vi "Run.vi"(8 "error in (no error)":errorcluster, 11 "DaqMx_Single in":refnum<class "DaqMx_Single.lvclass">) -> (0 "error out":errorcluster, 3 "DaqMx_Single out":refnum<class "DaqMx_Single.lvclass">)   [LabVIEW 2014, in "FgenPlugins.lvlib" / "DaqMx_Single.lvclass"]
uses:
  DaqMx_Single.lvclass
  FgenPluginBaseClass/FgenPluginsBase.lvclass/FgenPluginsBase.ctl
  FgenPluginBaseClass/Accessors/Read FunctionClass.vi
  FgenPluginBaseClass/Accessors/Write FunctionClass.vi
  FgenPluginBaseClass/Accessors/Read Channels.vi
  MemberClasses/FunctionBaseClass/FunctionBase.lvclass
  FgenPluginBaseClass/FgenPluginsBase.lvclass
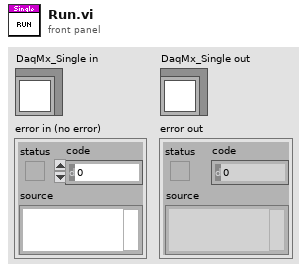
[diagram p1: front panel]
types:
  T1 = typedef "FgenPlugins.lvlib/DaqMx_Single.lvclass/clEvents.ctl" = cluster{"Stop":refnum<user-event>, "Params":refnum<user-event>}
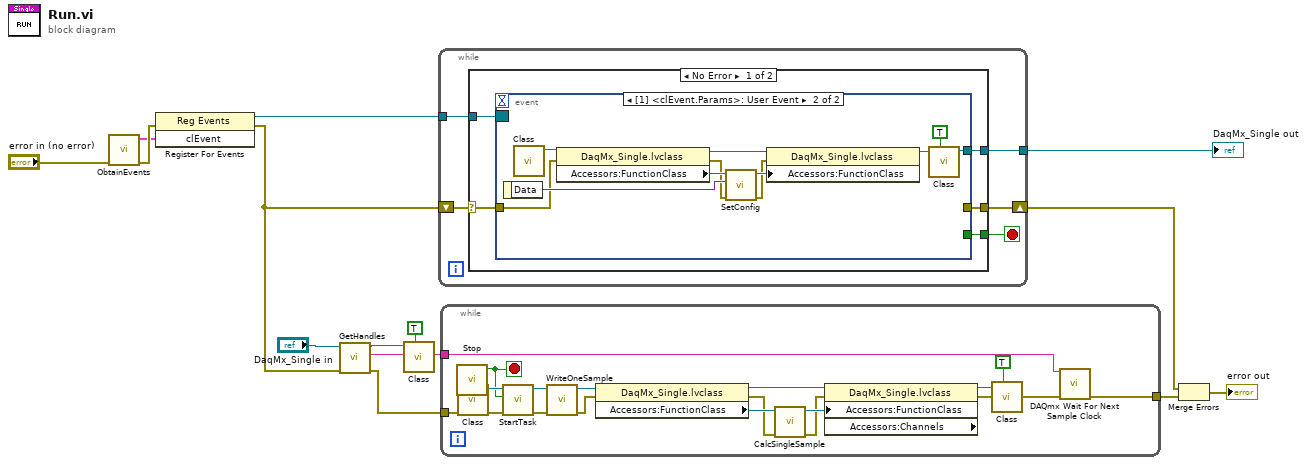
[diagram p0: block diagram]
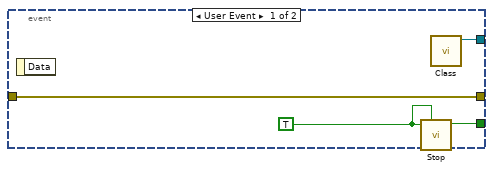
[diagram p2: hidden frame]
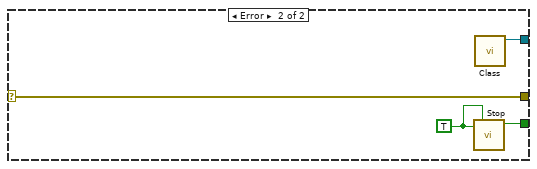
[diagram p3: hidden frame]
diagram:
  n1 = call "ObtainEvents.vi"("error in (no error)"="error in (no error)") -> ("error out"=w13:errorcluster, "clEvent"=w11:T1)  [unwired: 9 in]
  n2 = register-events(error in=w13, w11) -> (reference out=w14:refnum<event-registration>, error out=w2:errorcluster)  [unwired: 1 in]
  n3 = call "GetHandles.vi"("error in (no error)"=w2, "FgenPluginsBase in"="DaqMx_Single in") -> ("error out"=w1:errorcluster, "FirstHandle"=w3:string, "FgenPluginsBase out"=w4:refnum<class "DaqMx_Single.lvclass">)  [unwired: 6 in, 1 out]
  n4 = call "Class.vi"("Set? (f)"=TRUE, "DaqMx_Single in"=w4) -> ()  [unwired: 9 in, 1 out]
  n5 = while {
    tunnel: w14 -> [w19]
    tunnel: [w15] -> w10
    shift-right: [w16] -> w8
    shift-left: w2 -> [w17]
    stop <- w18 stop-if-true
    n6 = case shown="No Error" w17 {
      selector: w17 -> [w22 w41]
      tunnel: w19 -> [w24 _]
      tunnel: [w23 w42] -> w18
      tunnel: [w21 w41] -> w16
      tunnel: [w20 w40] -> w15
      frame No Error {
        n7 = event shown="[1] <clEvent.Params>: User Event" {
          selector: w24 -> [_ _]
          dyn-events: _ -> [_ _]
          timeout: _ -> [_ _]
          tunnel: [w27 _] -> w23
          tunnel: w22 -> [w26 w33]
          tunnel: [w26 _] -> w21
          tunnel: [w25 w29] -> w20
          event User Event {
            w28 = TRUE
            n8 = event-data() -> ()  [unwired: 1 in, 1 out]
            n9 = call "Stop.vi"("Set? (f)"=w28, "In"=w28) -> ("Out"=w27:bool)  [unwired: 9 in]
            n10 = call "Class.vi"() -> ("DaqMx_Single out"=w25:refnum<class "DaqMx_Single.lvclass">)  [unwired: 11 in]
          }
          event User Event {
            n11 = event-data() -> ("Data"=w37:variant)  [unwired: 1 in]
            n12 = call "Class.vi"() -> ("DaqMx_Single out"=w39:refnum<class "DaqMx_Single.lvclass">)  [unwired: 11 in]
            n13 = property class="DaqMx_Single.lvclass"(reference=w39, error in=w33) -> (reference out=w35:refnum<class "DaqMx_Single.lvclass">, error out=w32:errorcluster, "Accessors:FunctionClass"=w38:refnum<class "FunctionBase.lvclass">)
            n14 = call-dynamic "SetConfig.vi"("error in (no error)"=w32, "Variant"=w37, "FunctionBase in"=w38) -> ("error out"=w34:errorcluster, "FunctionBase out"=w36:refnum<class "FunctionBase.lvclass">)  [unwired: 7 in]
            n15 = property class="DaqMx_Single.lvclass"(reference=w35, error in=w34, "Accessors:FunctionClass"=w36) -> (reference out=w31:refnum<class "DaqMx_Single.lvclass">)  [unwired: 1 out]
            n16 = call "Class.vi"("Set? (f)"=TRUE, "DaqMx_Single in"=w31) -> ("DaqMx_Single out"=w29:refnum<class "DaqMx_Single.lvclass">)  [unwired: 9 in]
          }
        }
      }
      frame Error {
        w43 = TRUE
        n17 = call "Stop.vi"("Set? (f)"=w43, "In"=w43) -> ("Out"=w42:bool)  [unwired: 9 in]
        n18 = call "Class.vi"() -> ("DaqMx_Single out"=w40:refnum<class "DaqMx_Single.lvclass">)  [unwired: 11 in]
      }
    }
  }
  "DaqMx_Single out" <- w10
  n19 = while {
    tunnel: [w45] -> w7
    tunnel: w3 -> [w46]
    tunnel: w1 -> [w44]
    stop <- w48 stop-if-true
    n20 = call "Stop.vi"() -> ("Out"=w48:bool)  [unwired: 11 in]
    n21 = call "Class.vi"() -> ("DaqMx_Single out"=w49:refnum<class "DaqMx_Single.lvclass">)  [unwired: 11 in]
    n22 = call-dynamic "StartTask.vi"("error in (no error)"=w44, "Stop?"=w48, "DaqMx_Single in"=w49) -> ("error out"=w53:errorcluster, "DaqMx_Single out"=w52:refnum<class "DaqMx_Single.lvclass">)  [unwired: 7 in]
    n23 = call "WriteOneSample.vi"("error in (no error)"=w53, "DaqMx_Single in"=w52) -> ("error out"=w50:errorcluster, "DaqMx_Single out"=w51:refnum<class "DaqMx_Single.lvclass">)  [unwired: 8 in]
    n24 = property class="DaqMx_Single.lvclass"(reference=w51, error in=w50) -> (reference out=w58:refnum<class "DaqMx_Single.lvclass">, error out=w59:errorcluster, "Accessors:FunctionClass"=w60:refnum<class "FunctionBase.lvclass">)
    n25 = call-dynamic "CalcSingleSample.vi"("error in (no error)"=w59, "FunctionBase in"=w60) -> ("error out"=w56:errorcluster, "FunctionBase out"=w57:refnum<class "FunctionBase.lvclass">)  [unwired: 8 in]
    n26 = property class="DaqMx_Single.lvclass" props=["Accessors:FunctionClass", "Accessors:Channels"](reference=w58, error in=w56, "Accessors:FunctionClass"=w57) -> (reference out=w55:refnum<class "DaqMx_Single.lvclass">, error out=w47:errorcluster)  [unwired: 1 out]
    n27 = call "Class.vi"("Set? (f)"=TRUE, "DaqMx_Single in"=w55) -> ()  [unwired: 9 in, 1 out]
    n28 = call <vilib>:"DAQmx Wait For Next Sample Clock.vi"("task/channels in"=w46, "error in"=w47) -> ("error out"=w45:errorcluster)  [unwired: 11 in, 2 out]
  }
  n29 = Merge Errors(w8, w7) -> (→"error out":errorcluster)
